vi "Write DriveOutput.vi"(8 "error in (no error)":errorcluster, 10 "DriveOutput":T1 {"Control Mode" items=["PercentOutput"=0, "Position"=1, "Velocity"=2, "Current"=3, "Follower"=5, "MotionProfile"=6, "MotionMagic"=7, "MotionMagicArc"=8, "MotionProfileArc"=10, "Disabled"=15]}, 11 "DriveData in":refnum<class "DriveData.lvclass">) -> (0 "error out":errorcluster, 3 "DriveData out":refnum<class "DriveData.lvclass">)   [LabVIEW 2017]
uses:
  DriveData.lvclass
  R:/Documents/github/FRC4080/2018-robot-main/SubsystemData/SubsystemData.lvclass
  <vilib>/Rock Robotics/WPI/ThirdParty/Phoenix-LabVIEW/Motor Controller/Controls/CTRE_Phoenix_MotorControl_ControlMode.ctl
  DriveOutput.ctl
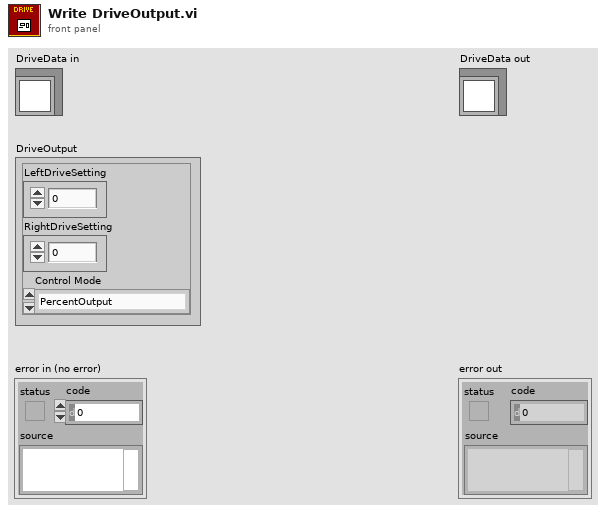
[diagram p1: front panel]
types:
  T1 = typedef "DriveData.lvclass/DriveOutput.ctl" = cluster{"LeftDriveSetting":dbl, "RightDriveSetting":dbl, "Control Mode":T2}
  T2 = typedef "CTRE_Phoenix_MotorControl_ControlMode.ctl" = u16
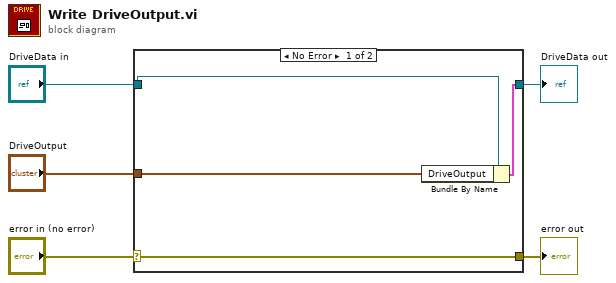
[diagram p0: block diagram]
diagram:
  n1 = case shown="No Error" "error in (no error)" {
    selector: "error in (no error)" -> [w9 w10]
    tunnel: [w9 w10] -> w4
    tunnel: [w7 w11] -> w2
    tunnel: "DriveData in" -> [w8 w11]
    tunnel: "DriveOutput" -> [w6 _]
    frame No Error {
      n2 = Bundle By Name(cluster=w8, "DriveOutput"=w6) -> (w7:cluster{})
    }
    frame Error {
    }
  }
  "error out" <- w4
  "DriveData out" <- w2
